vi "COOL32at.VI"() -> ()   [LabVIEW 2019]
panel:
  out "Waveform Graph":i32[](graph)
  out "Detector Y Pixels":i32
  in  "Shut Down":bool
  out "Raising Temperature":i32
  in  "Start Acquisition":bool
  out "Return  from Get Acquired Data":u32
  out "Detector X Pixels":i32
  out "Return from GetStatus":u32
  out "Return from Start Acquisition":u32
  out "Cooling":i32
  out "Return from SetTemperature":u32
  in  "Temperature":i32
  out "Return from CheckTimings":u32
  out "Calculated Exposure Value":sgl format="%.2f"
  in  "Exposure Time (secs)":sgl=0.05 format="%.2f"
  out "Return from Initialize":u32
  in  "Trigger":u32(ring) items=["Internal", "External"]
  # "Acquisition Mode: Single Scan\nReadout Mode: Full Vertical Binning\nCools to desired temperature, acquires data and then brings the temperature up to 0 in a controlled way."
  # "Status"
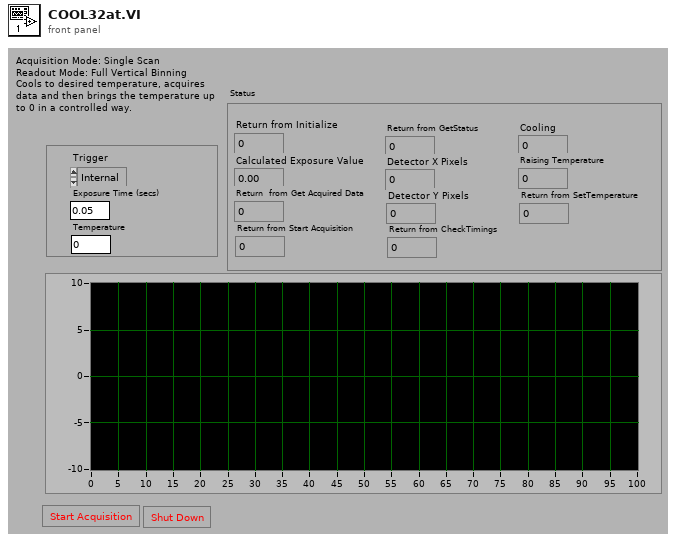
[diagram p1: front panel]
types:
  T1 = typedef "Error Code Enum typedef.ctl" = enum32{"N/A (0)", "DRV_ERROR_CODES", "DRV_SUCCESS", "DRV_VXDNOTINSTALLED", "DRV_ERROR_SCAN", "DRV_ERROR_CHECK_SUM", "DRV_ERROR_FILELOAD", "DRV_UNKNOWN_FUNC", "DRV_ERROR_VXD_INIT", "DRV_ERROR_ADDRESS", "DRV_ERROR_PAGELOCK", "DRV_ERROR_PAGEUNLOCK", "DRV_ERROR_BOARDTEST", "DRV_ERROR_ACK", "DRV_ERROR_UP_FIFO", "DRV_ERROR_PATTERN", "N/A (16)", "DRV_ACQUISITION_ERRORS", "DRV_ACQ_BUFFER", "DRV_ACQ_DOWNFIFO_FULL", "DRV_PROC_UNKONWN_INSTRUCTION", "DRV_ILLEGAL_OP_CODE", "DRV_KINETIC_TIME_NOT_MET", "DRV_ACCUM_TIME_NOT_MET", "DRV_NO_NEW_DATA", "N/A (25)", "DRV_SPOOLERROR", "N/A (27)", "N/A (28)", "N/A (29)", "N/A (30)", "N/A (31)", "N/A (32)", "DRV_TEMPERATURE_CODES", "DRV_TEMPERATURE_OFF", "DRV_TEMPERATURE_NOT_STABILIZED", "DRV_TEMPERATURE_STABILIZED", "DRV_TEMPERATURE_NOT_REACHED", "DRV_TEMPERATURE_OUT_RANGE", "DRV_TEMPERATURE_NOT_SUPPORTED", "DRV_TEMPERATURE_DRIFT", "N/A (41)", "N/A (42)", "N/A (43)", "N/A (44)", "N/A (45)", "N/A (46)", "N/A (47)", "N/A (48)", "DRV_GENERAL_ERRORS", "DRV_INVALID_AUX", "DRV_COF_NOTLOADED", "DRV_FPGAPROG", "DRV_FLEXERROR", "DRV_GPIBERROR", "N/A (55)", "N/A (56)", "N/A (57)", "N/A (58)", "N/A (59)", "N/A (60)", "N/A (61)", "N/A (62)", "N/A (63)", "DRV_DATATYPE", "DRV_DRIVER_ERRORS", "DRV_P1INVALID", "DRV_P2INVALID", "DRV_P3INVALID", "DRV_P4INVALID", "DRV_INIERROR", "DRV_COFERROR", "DRV_ACQUIRING", "DRV_IDLE", "DRV_TEMPCYCLE", "DRV_NOT_INITIALIZED", "DRV_P5INVALID", "DRV_P6INVALID", "DRV_INVALID_MODE", "DRV_INVALID_FILTER", "DRV_I2CERRORS", "DRV_I2CDEVNOTFOUND", "DRV_I2CTIMEOUT", "DRV_P7INVALID", "N/A (84)", "N/A (85)", "N/A (86)", "N/A (87)", "N/A (88)", "N/A (89)", "DRV_IOCERROR", "DRV_VRMVERSIONERROR"}
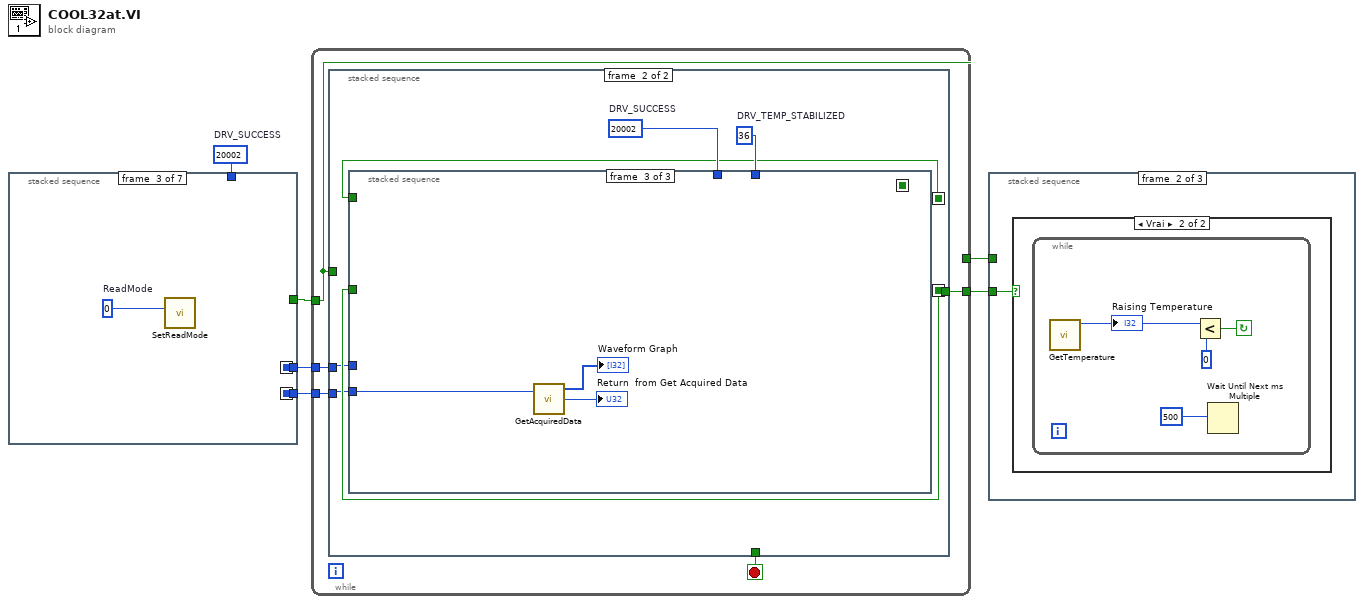
[diagram p0: block diagram]
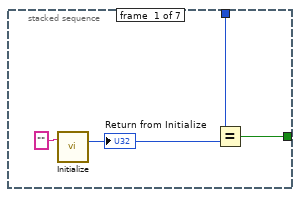
[diagram p2: hidden frame]
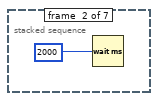
[diagram p3: hidden frame]
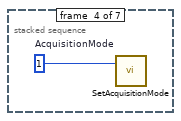
[diagram p4: hidden frame]
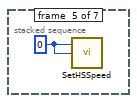
[diagram p5: hidden frame]
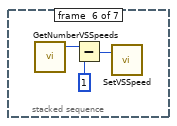
[diagram p6: hidden frame]
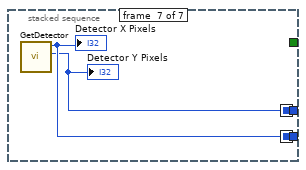
[diagram p7: hidden frame]
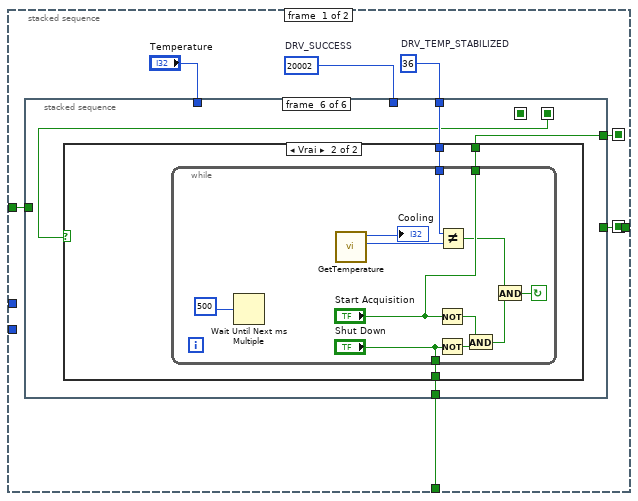
[diagram p8: hidden frame]
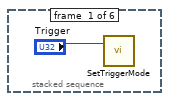
[diagram p9: hidden frame]
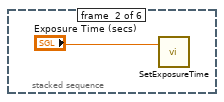
[diagram p10: hidden frame]
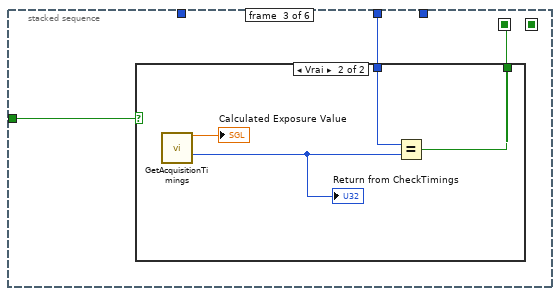
[diagram p11: hidden frame]
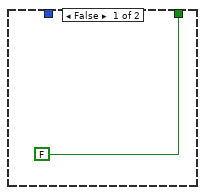
[diagram p12: hidden frame]
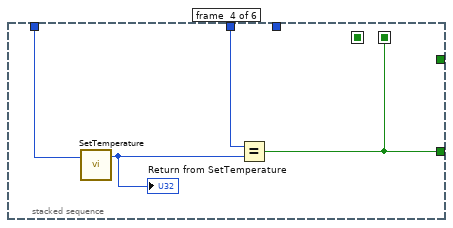
[diagram p13: hidden frame]
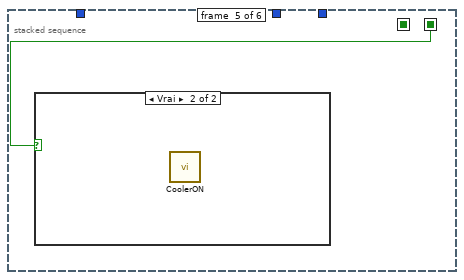
[diagram p14: hidden frame]
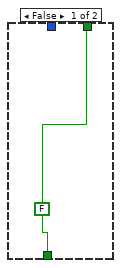
[diagram p16: hidden frame]
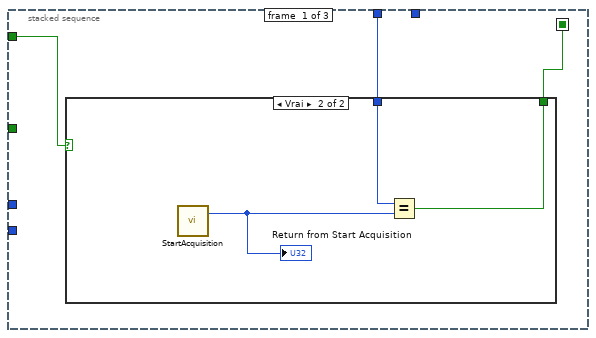
[diagram p17: hidden frame]
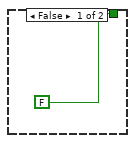
[diagram p18: hidden frame]
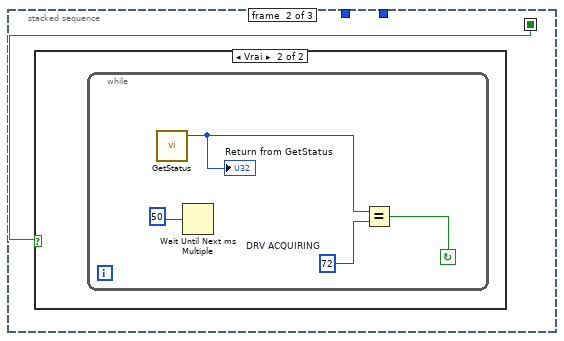
[diagram p19: hidden frame]
diagram:
  w4 = 20002  # DRV_SUCCESS
  n1 = stacked-sequence {
    seq-local: [_ _ _ _ _ _ w18] -> [_ _ _ _ _ _ _]
    seq-local: [_ _ _ _ _ _ w19] -> [_ _ _ _ _ _ _]
    tunnel: w4 -> [w8 _ _ _ _ _ _]
    tunnel: [w7 _ _ _ _ _ _] -> w3
    tunnel: [_ _ _ _ _ _ w18] -> w2
    tunnel: [_ _ _ _ _ _ w19] -> w1
    frame #0 {
      n2 = call <userlib>:"Initialize.vi"("directory (\"\")"="" ("directory (\"\")")) -> ("DLL error code"=w10:u32)  [unwired: 1 in, 1 out]
      "Return from Initialize" <- w10
      n3 = Equal?(x=w8, y=w10) -> (x = y?=w7:bool)
    }
    frame #1 {
      n4 = Wait (ms)(milliseconds to wait=u32 2000) -> ()  [unwired: 1 out]
    }
    frame #2 {
      w12 = u16 0  # ReadMode
      n5 = call <userlib>:"SetReadMode.vi"("mode"=w12) -> ()  [unwired: 1 in, 2 out]
    }
    frame #3 {
      w13 = u16 1  # AcquisitionMode
      n6 = call <userlib>:"SetAcquisitionMode.vi"("mode"=w13) -> ()  [unwired: 1 in, 2 out]
    }
    frame #4 {
      w14 = 0
      n7 = call <userlib>:"SetHSSpeed.vi"("index"=w14, "type"=w14) -> ()  [unwired: 2 in, 2 out]
    }
    frame #5 {
      n8 = call <userlib>:"GetNumberVSSpeeds.vi"() -> ("number"=w17:i32)  [unwired: 3 in, 2 out]
      n9 = Subtract(x=w17, y=1) -> (x-y=w15:i32)
      n10 = call <userlib>:"SetVSSpeed.vi"("index"=w15) -> ()  [unwired: 1 in, 2 out]
    }
    frame #6 {
      n11 = call <userlib>:"GetDetector.vi"() -> ("ypixels"=w18:i32, "xpixels"=w19:i32)  [unwired: 4 in, 2 out]
      "Detector Y Pixels" <- w18
      "Detector X Pixels" <- w19
    }
  }
  n12 = while {
    tunnel: [w20] -> w6
    tunnel: [w24] -> w5
    tunnel: w3 -> [w20]
    tunnel: w2 -> [w23]
    tunnel: w1 -> [w22]
    stop <- w21 stop-if-true
    n13 = stacked-sequence {
      seq-local: [w31 _] -> [_ w69]
      seq-local: [w30 _] -> [_ w68]
      tunnel: [_ w68] -> w24
      tunnel: w23 -> [_ w67]
      tunnel: w22 -> [_ w66]
      tunnel: [w26 _] -> w21
      tunnel: w20 -> [w25 _]
      frame #0 {
        w27 = 36  # DRV_TEMP_STABILIZED
        w29 = 20002  # DRV_SUCCESS
        n14 = stacked-sequence {
          seq-local: [_ _ w34 _ _ _] -> [_ _ _ _ _ _]
          seq-local: [_ _ _ w42 _ _] -> [_ _ _ _ w46 w49]
          tunnel: w29 -> [_ _ w36 w45 _ _]
          tunnel: "Temperature" -> [_ _ _ w43 _ _]
          tunnel: w27 -> [_ _ _ _ _ w50]
          tunnel: [_ _ _ _ _ w47] -> w31
          tunnel: [_ _ _ w42 _ _] -> w30
          tunnel: [_ _ _ _ _ w48] -> w26
          tunnel: w25 -> [_ _ w35 _ _ _]
          frame #0 {
            n15 = call <userlib>:"SetTriggerMode.vi"("mode"="Trigger") -> ()  [unwired: 1 in, 2 out]
          }
          frame #1 {
            n16 = call <userlib>:"SetExposureTime.vi"("time"="Exposure Time (secs)") -> ()  [unwired: 1 in, 2 out]
          }
          frame #2 {
            n17 = case shown="Vrai" w35 {
              tunnel: w36 -> [_ w39]
              tunnel: [FALSE w41] -> w34
              frame False {
              }
              frame True {
                n18 = call <userlib>:"GetAcquisitionTimings.vi"() -> ("exposure"=→"Calculated Exposure Value":sgl, "DLL error code"=w38:u32)  [unwired: 11 in, 3 out]
                "Return from CheckTimings" <- w38
                n19 = Equal?(x=w39, y=w38) -> (x = y?=w41:bool)
              }
            }
          }
          frame #3 {
            n20 = call <userlib>:"SetTemperature.vi"("temperature"=w43) -> ("DLL error code"=w44:u32)  [unwired: 1 in, 1 out]
            "Return from SetTemperature" <- w44
            n21 = Equal?(x=w45, y=w44) -> (x = y?=w42:bool)
          }
          frame #4 {
            n22 = case shown="Vrai" w46 {
              frame False {
              }
              frame True {
                n23 = call <userlib>:"CoolerON.vi"() -> ()  [unwired: 2 in, 2 out]
              }
            }
          }
          frame #5 {
            n24 = case shown="Vrai" w49 {
              tunnel: w50 -> [_ w54]
              tunnel: [w51 w53] -> w48
              tunnel: [w51 w52] -> w47
              frame False {
                w51 = FALSE
              }
              frame True {
                n25 = while {
                  tunnel: w54 -> [w64]
                  tunnel: ["Shut Down"] -> w53
                  tunnel: ["Start Acquisition"] -> w52
                  stop <- w57 continue-if-true
                  n26 = Wait Until Next ms Multiple(millisecond multiple=u32 500) -> ()  [unwired: 1 out]
                  n27 = call <userlib>:"GetTemperature.vi"() -> ("status"=w62:T1, "temperature"=→"Cooling":i32)  [unwired: 4 in, 2 out]
                  n28 = Not(x="Start Acquisition") -> (.not. x?=w59:bool)
                  n29 = Not(x="Shut Down") -> (.not. x?=w61:bool)
                  n30 = Not Equal?(x=w64, y=w62) -> (x != y?=w56:bool)
                  n31 = And(x=w59, y=w61) -> (x .and. y?=w55:bool)
                  n32 = And(x=w56, y=w55) -> (x .and. y?=w57:bool)
                }
              }
            }
          }
        }
      }
      frame #1 {
        w70 = 36  # DRV_TEMP_STABILIZED
        w71 = 20002  # DRV_SUCCESS
        n33 = stacked-sequence {
          seq-local: [w73 _ _] -> [_ w79 _]
          tunnel: w71 -> [w74 _ _]
          tunnel: w70 -> [_ _ _]
          tunnel: w69 -> [w72 _ _]
          tunnel: w68 -> [_ _ _]
          tunnel: w67 -> [_ _ _]
          tunnel: w66 -> [_ _ w85]
          frame #0 {
            n34 = case shown="Vrai" w72 {
              tunnel: [FALSE w78] -> w73
              tunnel: w74 -> [_ w77]
              frame False {
              }
              frame True {
                n35 = call <userlib>:"StartAcquisition.vi"() -> ("DLL error code"=w76:u32)  [unwired: 2 in, 1 out]
                "Return from Start Acquisition" <- w76
                n36 = Equal?(x=w77, y=w76) -> (x = y?=w78:bool)
              }
            }
          }
          frame #1 {
            n37 = case shown="Vrai" w79 {
              frame False {
              }
              frame True {
                n38 = while {
                  stop <- w82 continue-if-true
                  w81 = u16 72  # DRV ACQUIRING
                  n39 = call <userlib>:"GetStatus.vi"() -> ("status"=w80:T1)  [unwired: 3 in, 2 out]
                  "Return from GetStatus" <- w80
                  n40 = Wait Until Next ms Multiple(millisecond multiple=u32 50) -> ()  [unwired: 1 out]
                  n41 = Equal?(x=w80, y=w81) -> (x = y?=w82:bool)
                }
              }
            }
          }
          frame #2 {
            n42 = call <userlib>:"GetAcquiredData.vi"("size"=w85) -> ("DLL error code"=→"Return  from Get Acquired Data":u32, "array"=→"Waveform Graph":i32[])  [unwired: 2 in, 1 out]
          }
        }
      }
    }
  }
  n43 = stacked-sequence {
    tunnel: w5 -> [_ w87 _]
    tunnel: w6 -> [_ _ w92]
    frame #0 {
      n44 = call <userlib>:"CoolerOFF.vi"() -> ()  [unwired: 2 in, 2 out]
    }
    frame #1 {
      n45 = case shown="Vrai" w87 {
        frame False {
        }
        frame True {
          n46 = while {
            stop <- w90 continue-if-true
            n47 = call <userlib>:"GetTemperature.vi"() -> ("temperature"=w89:i32)  [unwired: 4 in, 3 out]
            "Raising Temperature" <- w89
            n48 = Less?(x=w89, y=i16 0) -> (x < y?=w90:bool)
            n49 = Wait Until Next ms Multiple(millisecond multiple=u32 500) -> ()  [unwired: 1 out]
          }
        }
      }
    }
    frame #2 {
      n50 = case shown="Vrai" w92 {
        frame False {
        }
        frame True {
          n51 = call <userlib>:"ShutDown.vi"() -> ()  [unwired: 2 in, 2 out]
        }
      }
    }
  }
